vi "Init.vi"(8 "error in (no error)":errorcluster, 11 "XY Stage Class in":refnum<class "XY Stage Class.lvclass">) -> (0 "error out":errorcluster, 3 "XY Stage Class out":refnum<class "XY Stage Class.lvclass">)   [LabVIEW 2022 SP3, in "XY Stage Class.lvclass"]
uses:
  XY Stage Class.lvclass
  XY Stage Class.lvclass/XY Stage Class.ctl
  iView/base view/base view.lvclass
  XY Controller/XY Stage Controller/XY Stage Controller.lvclass
  data.ctl
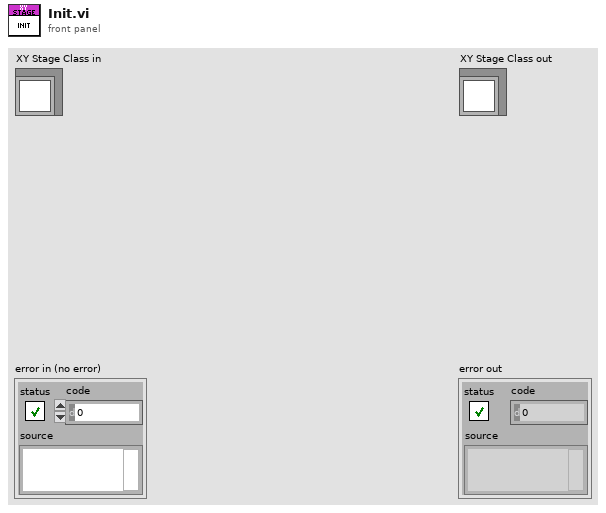
[diagram p1: front panel]
types:
  T1 = typedef "XY Stage Class.lvclass/data.ctl" = cluster{"XY Stage Controller":refnum<class "XY Stage Controller.lvclass">}
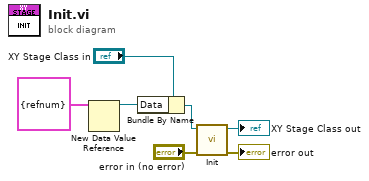
[diagram p0: block diagram]
diagram:
  n1 = New Data Value Reference(data value=T1 {"XY Stage Controller"=refnum} ("Data")) -> (data value reference=w1:refnum<data-value>)  [unwired: 1 in, 1 out]
  n2 = Bundle By Name(cluster="XY Stage Class in", "Data"=w1) -> (w2:refnum<class "XY Stage Class.lvclass">)
  n3 = call-parent "Init.vi"("error in (no error)"="error in (no error)", "base view in"=w2) -> ("error out"=→"error out":errorcluster, "base view out"=→"XY Stage Class out":refnum<class "XY Stage Class.lvclass">)  [unwired: 8 in]
